vi "Read Line Followers.vi"(8 "error in":errorcluster, 11 "TeleOp Data Cluster in":T1) -> (0 "error out":errorcluster, 3 "Teleop Data Cluster out":T1)   [LabVIEW 2018]
uses:
  TypeDefs/Teleop Data Cluster.ctl
  TypeDefs/typedef_enum_Refnums.ctl
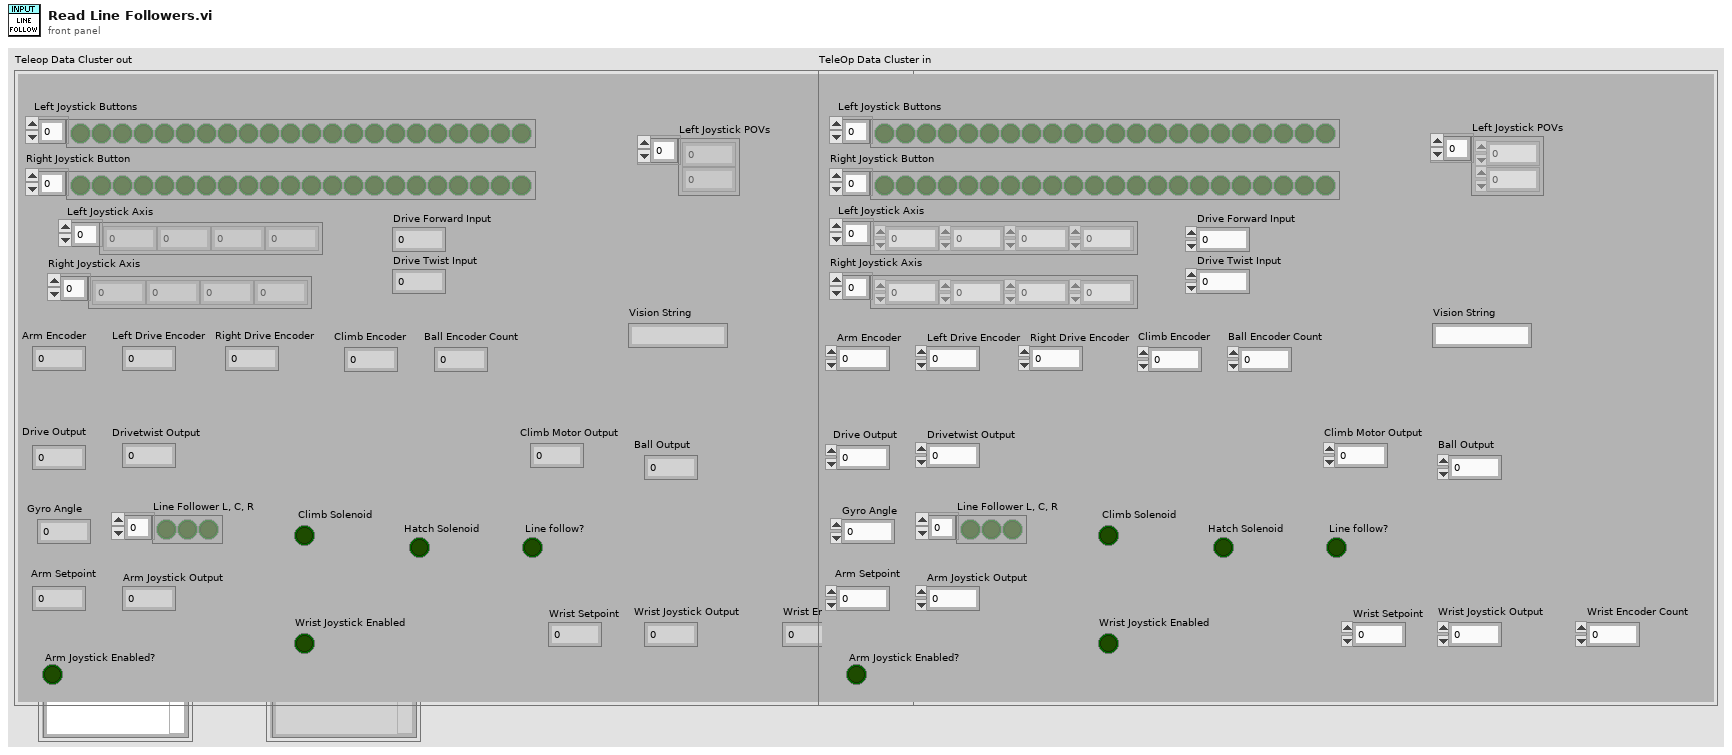
[diagram p1: front panel]
types:
  T1 = typedef "Teleop Data Cluster.ctl" = cluster{"Drive Forward Input ":dbl, "Drive Twist Input":dbl, "Drive Output":dbl, "Drivetwist Output":dbl, "Left Joystick Buttons":bool[], "Left Joystick Axis":dbl[], "Right Joystick Axis":dbl[], "Right Joystick Button":bool[], "Arm Encoder":dbl, "Left Drive Encoder":dbl, "Right Drive Encoder":dbl, "Gyro Angle ":dbl, "Arm Joystick Output  ":dbl, "Line Follower L, C, R ":bool[], "Line follow?":bool, " Climb Solenoid":bool, "Wrist Encoder Count":dbl, "Wrist Joystick Output":dbl, "Ball Encoder Count":dbl, "Ball Output":dbl, "Climb Encoder":dbl, "Climb Motor Output":dbl, " Hatch Solenoid":bool, "Arm Setpoint ":dbl, "Wrist Setpoint ":dbl, "Arm Joystick Enabled?":bool, "Wrist Joystick Enabled":bool, "Vision String":string, "Left Joystick POVs":i16[]}
  T2 = typedef "typedef_enum_Refnums.ctl" = enum16{"Ball_Encoder", "Ball_Motor", "Camera", "Linefollow_3", "Linefollow_2", "Linefollow_1", "Gyro", "Hatch_Solenoid", "Climb_Back_Solenoid", "Arm_Encoder", "Arm_Motor", "Lift_Encoder", "Drive", "Drive_Motor_R", "Drive_Motor_L", "Drive_Encoder_R", "Drive_Encoder_L", "Joy_R", "Joy_L", "Wrist_Motor", "Wrist_Encoder", "Climb Upper Limit", "Climb Lower Limit ", "Climb_Front_Motor"}
  T3 = typedef "WPI_DigitalInputDevRef.ctl" = cluster{"DevStatus":errorcluster, "DIO Channel":T4}
  T4 = typedef "FPGA_DIOChannel.ctl" = enum8{"DIO 0", "DIO 1", "DIO 2", "DIO 3", "DIO 4", "DIO 5", "DIO 6", "DIO 7", "DIO 8", "DIO 9", "DIO MXP 0", "DIO MXP 1", "DIO MXP 2", "DIO MXP 3", "DIO MXP 4", "DIO MXP 5", "DIO MXP 6", "DIO MXP 7", "DIO MXP 8", "DIO MXP 9", "DIO MXP 10", "DIO MXP 11", "DIO MXP 12", "DIO MXP 13", "DIO MXP 14", "DIO MXP 15", "SPI Port CS1", "SPI Port CS2", "SPI Port CS3", "SPI Port MISO", "SPI Port MOSI", "Invalid"}
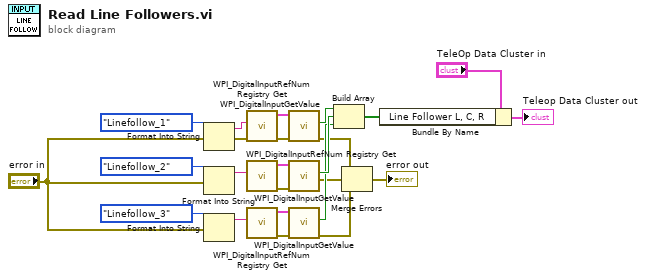
[diagram p0: block diagram]
diagram:
  n1 = Format Into String(error in="error in", typedef_enum_Refnums."Linefollow_1" ("RefNums")) -> (resulting string=w7:string, error out=w13:errorcluster)  [unwired: 2 in]
  n2 = Format Into String(error in="error in", typedef_enum_Refnums."Linefollow_2" ("RefNums")) -> (resulting string=w9:string)  [unwired: 2 in, 1 out]
  n3 = Format Into String(error in="error in", typedef_enum_Refnums."Linefollow_3" ("RefNums")) -> (resulting string=w11:string)  [unwired: 2 in, 1 out]
  n4 = call <vilib>:"WPI_DigitalInputRefNum Registry Get.vi"("error in (no error)"=w13, "refnum name"=w7) -> ("error out"=w18:errorcluster, "DigitalInputDevRef"=w19:T3)  [unwired: 8 in]
  n5 = call <vilib>:"WPI_DigitalInputRefNum Registry Get.vi"("refnum name"=w9) -> ("error out"=w16:errorcluster, "DigitalInputDevRef"=w17:T3)  [unwired: 9 in]
  n6 = call <vilib>:"WPI_DigitalInputRefNum Registry Get.vi"("refnum name"=w11) -> ("error out"=w15:errorcluster, "DigitalInputDevRef"=w14:T3)  [unwired: 9 in]
  n7 = call <vilib>:"WPI_DigitalInputGetValue.vi"("error in (no error)"=w18, "DigitalInputDevRef"=w19) -> ("error out"=w5:errorcluster, "Value"=w23:bool)  [unwired: 7 in, 1 out]
  n8 = call <vilib>:"WPI_DigitalInputGetValue.vi"("error in (no error)"=w16, "DigitalInputDevRef"=w17) -> ("error out"=w4:errorcluster, "Value"=w21:bool)  [unwired: 7 in, 1 out]
  n9 = call <vilib>:"WPI_DigitalInputGetValue.vi"("error in (no error)"=w15, "DigitalInputDevRef"=w14) -> ("error out"=w3:errorcluster, "Value"=w20:bool)  [unwired: 7 in, 1 out]
  n10 = Build Array(w23, w21, w20) -> (w22:bool[])
  n11 = Merge Errors(w5, w4, w3) -> (→"error out":errorcluster)
  n12 = Bundle By Name(cluster="TeleOp Data Cluster in", "Line Follower L, C, R"=w22) -> (→"Teleop Data Cluster out":T1)
